vi "DSF.Engine.Pool.Write FIFO.vi"(8 "error in (no error)":errorcluster, 9 "timeout in ms (0)":i32 format="%d ms", 10 "element":i32, 11 "Pool in":refnum<class "DSF.Engine.Pool.lvclass">) -> (0 "error out":errorcluster, 1 "timed out?":bool, 3 "Pool out":refnum<class "DSF.Engine.Pool.lvclass">)   [LabVIEW 2016, in "DSF.Engine.lvlib" / "DSF.Engine.Pool.lvclass"]
uses:
  DSF.Engine.Pool.lvclass
  DSF.Engine.Pool.lvclass/DSF.Engine.Pool.ctl
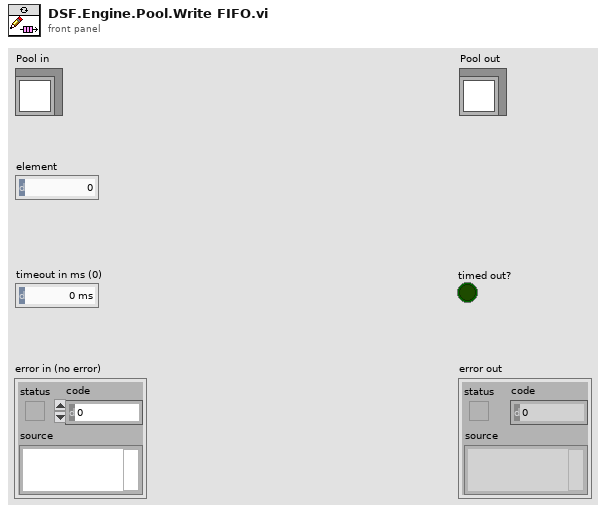
[diagram p1: front panel]
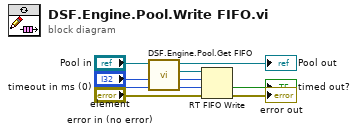
[diagram p0: block diagram]
diagram:
  n1 = call "DSF.Engine.Pool.Get FIFO.vi"("Pool in"="Pool in") -> ("FIFO"=w6:refnum<k33>, "Pool out"=→"Pool out":refnum<class "DSF.Engine.Pool.lvclass">)  [unwired: 9 in]
  n2 = RT FIFO Write(0:w6, 1:"element", 2:"timeout in ms (0)", 3:"error in (no error)") -> (10:→"timed out?":bool, 11:→"error out":errorcluster)  [unwired: 1 in, 2 out]
